vi "Write Commit Operation Errors.vi"(8 "Error In":errorcluster, 10 "Commit Operation Errors":errorcluster, 11 "Commit in":refnum<class "Commit.lvclass">) -> (0 "Error Out":errorcluster, 3 "Commit out":refnum<class "Commit.lvclass">)   [LabVIEW 2017, in "CL_G3_VIComponentBuilder.lvlib" / "Commit.lvclass"]
uses:
  Commit.lvclass
  Commit.lvclass/Commit.ctl
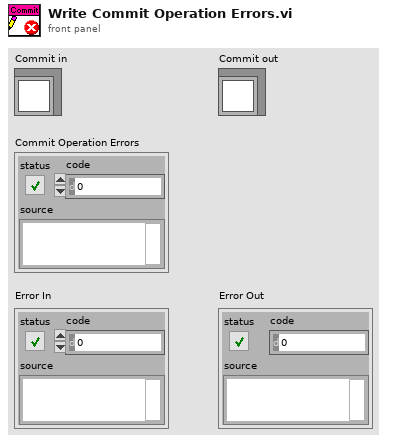
[diagram p1: front panel]
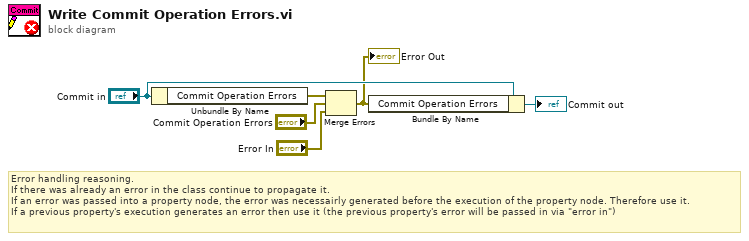
[diagram p0: block diagram]
diagram:
  # "Error handling reasoning.\nIf there was already an error in the class continue to propagate it.\nIf an error was passed into a property node, the error was necessairly generated before the execution of the property node. Therefore use it.\nIf a previous property's execution generates an error then use it (the previous property's error will be passed in via \"error in\")"
  n1 = Unbundle By Name("Commit in") -> ("Commit Operation Errors"=w4:errorcluster)
  n2 = Merge Errors(w4, "Commit Operation Errors", "Error In") -> (w1:errorcluster)
  "Error Out" <- w1
  n3 = Bundle By Name(cluster="Commit in", "Commit Operation Errors"=w1) -> (→"Commit out":refnum<class "Commit.lvclass">)
